vi "GetEventsFromDatabase.vi"() -> ()   [LabVIEW 2020]
uses:
  settingsManagement/DataBaseInterface/Controls/DataBaseOptions.ctl
  settingsManagement/DataBaseInterface/Controls/DataBaseAuthentication.ctl
  <vilib>/SAPHIR/GDataBase for MySQL(tm)/MySQL/MySQLConnector.lvclass/MySQLConnector.ctl
  <vilib>/SAPHIR/GDataBase for MySQL(tm)/NetworkStream/MySQLNetworkStream.lvclass/MySQLNetworkStream.ctl
  settingsManagement/DataBaseInterface/Private/GetMySQL_RT_Object.vi
  <vilib>/SAPHIR/GDataBase for MySQL(tm)/NetworkStream/public/SendCommand.vi
  <vilib>/SAPHIR/GDataBase for MySQL(tm)/NetworkStream/public/locker/AcquireLocker.vi
  <vilib>/SAPHIR/GDataBase for MySQL(tm)/NetworkStream/public/locker/ReleaseLocker.vi
  <vilib>/SAPHIR/GDataBase for MySQL(tm)/NetworkStream/public/WritePacket.vi
  <vilib>/SAPHIR/GDataBase for MySQL(tm)/MySQL/public/Open.vi
  <vilib>/Utility/error.llb/Trim Whitespace.vi
  <vilib>/Utility/semaphor.llb/Acquire Semaphore.vi
  <vilib>/SAPHIR/GDataBase for MySQL(tm)/NetworkStream/public/ReadResultPacket.vi
  <vilib>/Utility/semaphor.llb/Release Semaphore.vi
  <vilib>/SAPHIR/GDataBase for MySQL(tm)/MySQL/MySQLConnector.lvclass
  settingsManagement/DataBaseInterface/DataBaseInterface.lvlib
panel:
  out "String":string
  out "Query Results out":string[][](array[string])
  out "error out":errorcluster
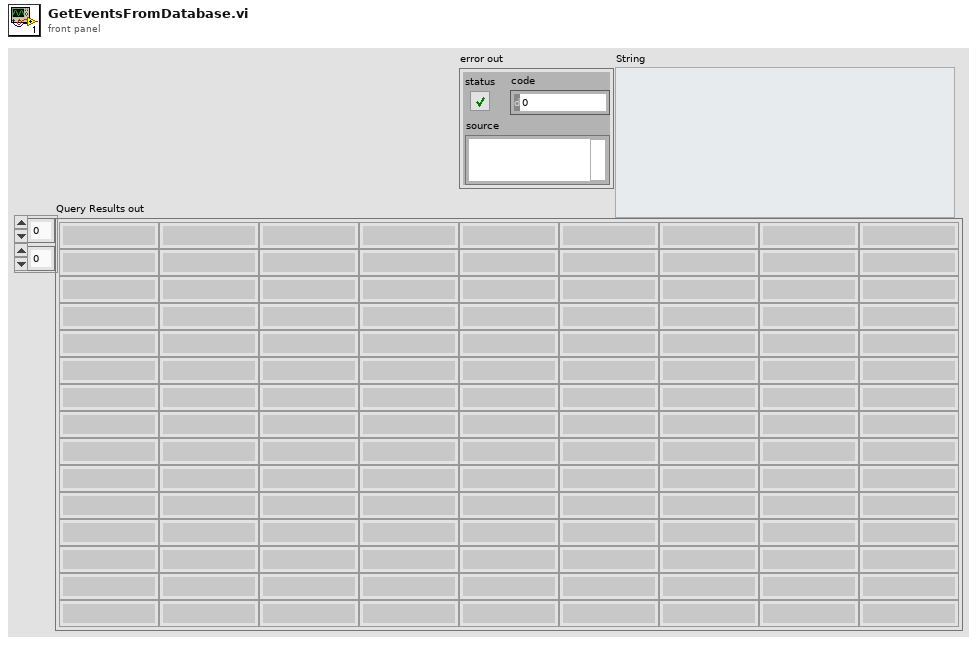
[diagram p1: front panel]
types:
  T1 = typedef "DataBaseInterface.lvlib/DataBaseAuthentication.ctl" = cluster{"username":string, "password":string, "database":string}
  T2 = typedef "DataBaseInterface.lvlib/DataBaseOptions.ctl" = cluster{"Timeout":u32, "Read Timeout":u32, "Auto Reconnect":bool}
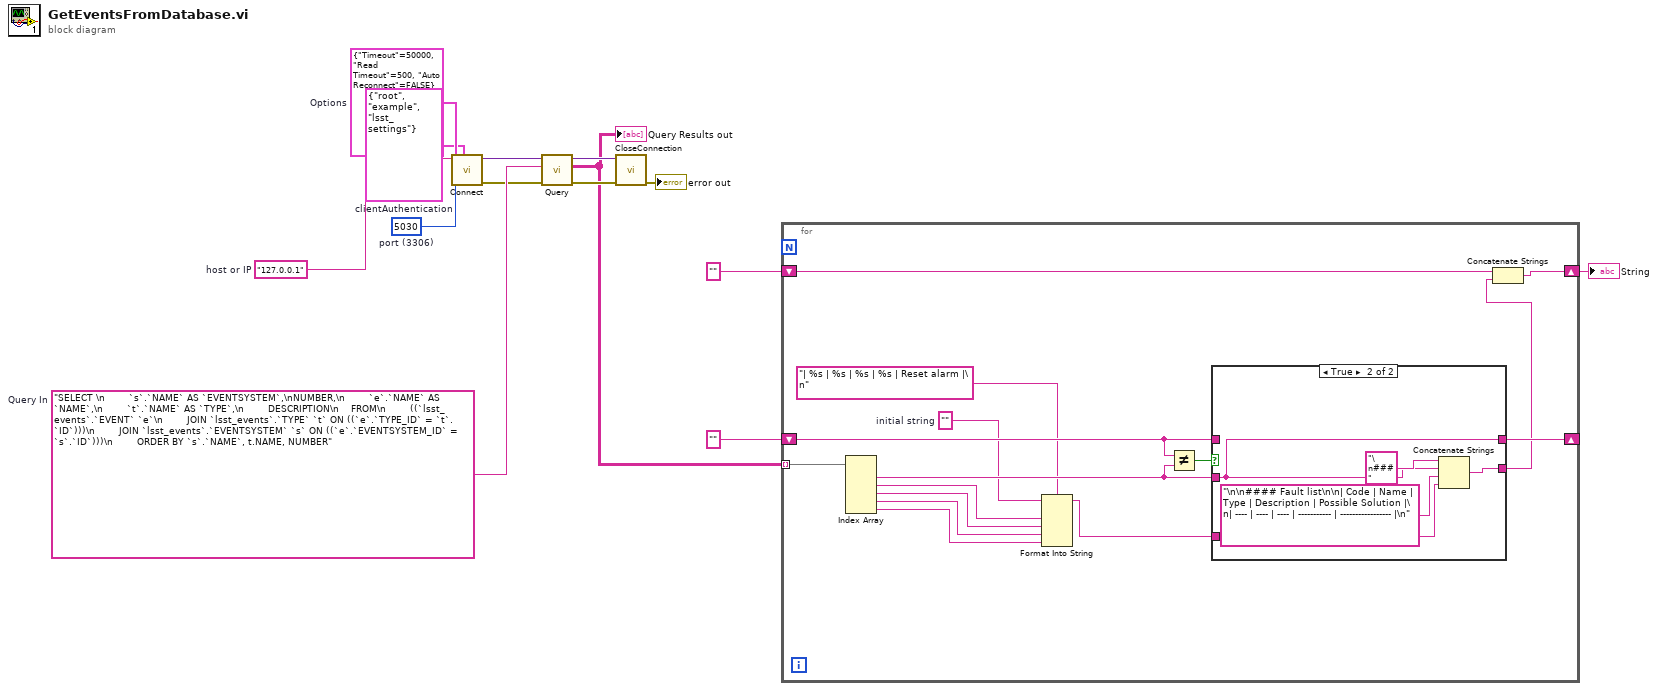
[diagram p0: block diagram]
diagram:
  w5 = u16 5030  # port (3306)
  w6 = T1 {"username"="root", "password"="example", "database"="lsst_settings"}  # clientAuthentication
  w7 = T2 {"Timeout"=50000, "Read Timeout"=500, "Auto Reconnect"=FALSE}  # Options
  w8 = "127.0.0.1"  # host or IP
  w14 = "SELECT \n        `s`.`NAME` AS `EVENTSYSTEM`,\nNUMBER,\n        `e`.`NAME` AS `NAME`,\n        `t`.`NAME` AS `TYPE`,\n        DESCRIPTION\n    FROM\n        ((`lsst_events`.`EVENT` `e`\n        JOIN `lsst_events`.`TYPE` `t` ON ((`e`.`TYPE_ID` = `t`.`ID`)))\n        JOIN `lsst_events`.`EVENTSYSTEM` `s` ON ((`e`.`EVENTSYSTEM_ID` = `s`.`ID`)))\n        ORDER BY `s`.`NAME`, t.NAME, NUMBER"  # Query In
  n1 = call "Connect.vi"("clientAuthentication"=w6, "Options"=w7, "port (3306)"=w5, "host or IP"=w8) -> ("error out"=w11:errorcluster, "DatabaseObject out"=w13:variant)  [unwired: 6 in]
  n2 = call <vilib>:"Query.vi"("error in (no error)"=w11, "Query In"=w14, "DataBase Object"=w13) -> ("error out"=w10:errorcluster, "Query Results out"=w4:string[][], "DataBase Object out"=w12:variant)  [unwired: 6 in]
  "Query Results out" <- w4
  n3 = call "CloseConnection.vi"("error in (no error)"=w10, "DataBase Object"=w12) -> ("error out"=→"error out":errorcluster)  [unwired: 9 in]
  n4 = for {
    tunnel: w4 -> [w27] mode=indexing
    shift-right: [w28] -> w1
    shift-left: "" -> [w29]
    shift-right: [w25] -> _
    shift-left: "" -> [w23]
    w20 = ""  # initial string
    n5 = Index Array(array=w27) -> (element #1=w24:string, element #2=w19:string, element #3=w18:string, element #4=w17:string, element #5=w16:string)  [unwired: 5 in]
    n6 = Format Into String(format string="| %s | %s | %s | %s | Reset alarm |\n", initial string=w20, w19, w18, w17, w16) -> (resulting string=w15:string)  [unwired: 1 in, 1 out]
    n7 = Not Equal?(x=w23, y=w24) -> (x != y?=w26:bool)
    n8 = case shown="True" w26 {
      tunnel: [w31 w35] -> w25
      tunnel: w24 -> [_ w35]
      tunnel: w23 -> [w31 _]
      tunnel: [w30 w33] -> w22
      tunnel: w15 -> [w30 w32]
      frame False {
      }
      frame True {
        n9 = Concatenate Strings("\n### ", w35, "\n\n#### Fault list\n\n| Code | Name | Type | Description | Possible Solution |\n| ---- | ---- | ---- | ----------- | ----------------- |\n", w32) -> (w33:string)
      }
    }
    n10 = Concatenate Strings(w29, w22) -> (w28:string)
  }
  "String" <- w1
